vi "Observe Data.vi"(6 "Time Stamp":timestamp, 8 "error in (no error)":errorcluster, 9 "Value":variant, 10 "Datum Name":string, 11 "IObserver in":refnum<class "IObserver.lvclass">) -> (0 "error out":errorcluster, 3 "IObserver out":refnum<class "IObserver.lvclass">)   [LabVIEW 2018, in "MVA Framework.lvlib" / "IObserver.lvlib" / "IObserver.lvclass"]
doc: "观察数据"
uses:
  IObserver.lvclass
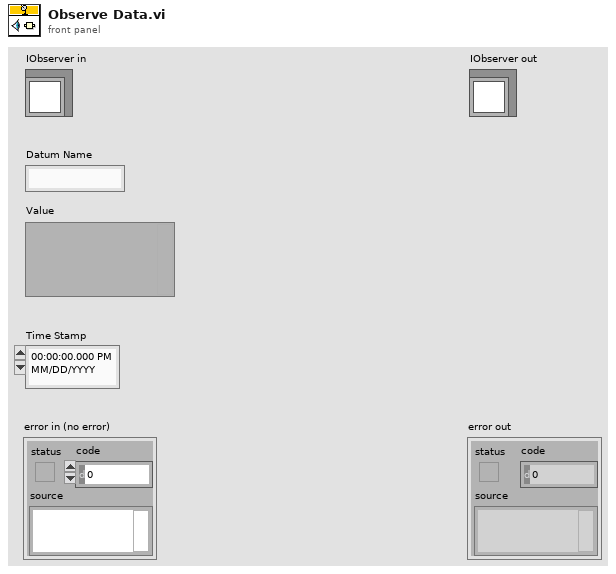
[diagram p1: front panel]
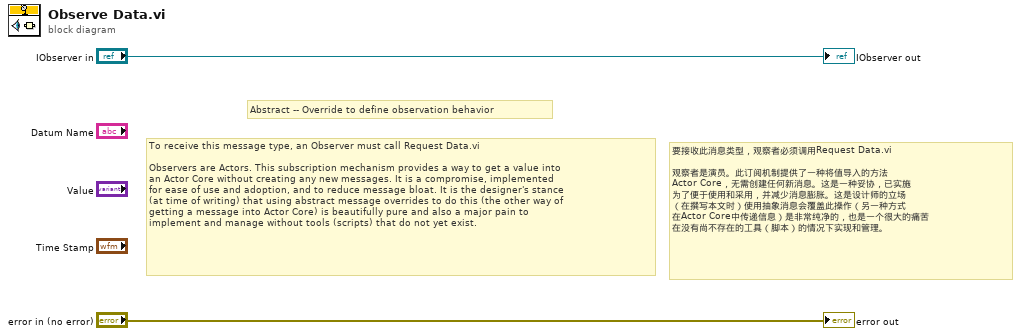
[diagram p0: block diagram]
diagram:
  # "要接收此消息类型，观察者必须调用Request Data.vi\n\n观察者是演员。此订阅机制提供了一种将值导入的方法\nActor Core，无需创建任何新消息。这是一种妥协，已实施\n为了便于使用和采用，并减少消息膨胀。这是设计师的立场\n（在撰写本文时）使用抽象消息会覆盖此操作（另一种方式\n在Actor Core中传递信息）是非常纯净的，也是一个很大的痛苦\n在没有尚不存在的工具（脚本）的情况下实现和管理。"
  # "To receive this message type, an Observer must call Request Data.vi\n\nObservers are Actors. This subscription mechanism provides a way to get a value into\nan Actor Core without creating any new messages. It is a compromise, implemented\nfor ease of use and adoption, and to reduce message bloat. It is the designer's stance\n(at time of writing) that using abstract message overrides to do this (the other way of\ngetting a message into Actor Core) is beautifully pure and also a major pain to\nimplement and manage without tools (scripts) that do not yet exist."
  # "Abstract -- Override to define observation behavior"
  "error out" <- "error in (no error)"
  "IObserver out" <- "IObserver in"
